vi "Cache Message.vi"(10 "Message":T1={"Source"="", "Destination"="", "Time Stamp"=timestamp(0 s since 1904-01-01), "Command"="", "Data"=variant(string "")}, 11 "Message History In":string[][](array[string])) -> (3 "Message History Out":string[][](array[string]))   [LabVIEW 2020, in "RxnRover.lvlib"]
uses:
  RxnRover.lvlib
  <userlib>/RxnRover/DynamicReentrant/src/Type Defs/Message.ctl
  <userlib>/RxnRover/DynamicReentrant/Dynamic Reentrant.lvlib
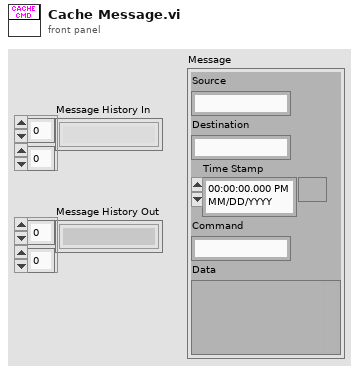
[diagram p1: front panel]
types:
  T1 = typedef "Dynamic Reentrant.lvlib/Message.ctl" = cluster{"Source":string, "Destination":string, "Time Stamp":timestamp, "Command":string, "Data":variant}
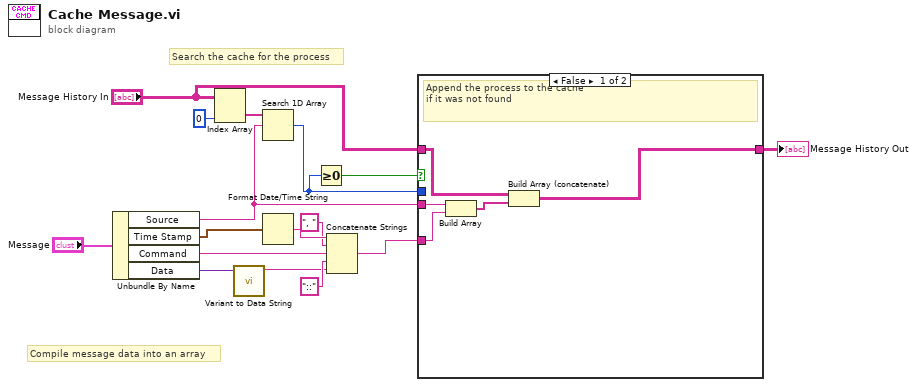
[diagram p0: block diagram]
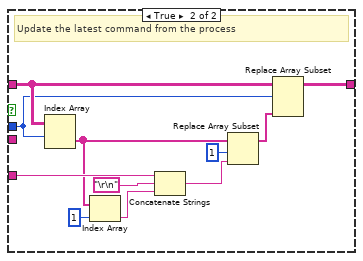
[diagram p2: hidden frame]
diagram:
  # "Search the cache for the process"
  # "Compile message data into an array"
  n1 = Unbundle By Name("Message") -> ("Source"=w3:string, "Time Stamp"=w9:timestamp, "Command"=w8:string, "Data"=w1:variant)
  n2 = Index Array(array="Message History In", index (col)=0 ("disabled index (col)")) -> (element=w16:string[])  [unwired: 1 in]
  n3 = call "Variant to Data String.vi"("Data"=w1) -> ("string"=w2:string)  [unwired: 9 in, 1 out]
  n4 = Search 1D Array(1D array=w16, element=w3) -> (index of element=w10:i32)  [unwired: 1 in]
  n5 = Format Date/Time String(seconds (now)=w9) -> (date/time string=w7:string)  [unwired: 2 in]
  n6 = Greater Or Equal To 0?(x=w10) -> (x >= 0?=w14:bool)
  n7 = Concatenate Strings(w7, ", " ("string"), w8, "::" ("string"), w2) -> (w4:string)
  n8 = case shown="False" w14 {
    tunnel: w10 -> [_ w27]
    tunnel: [w20 w26] -> w12
    tunnel: "Message History In" -> [w21 w28]
    tunnel: w4 -> [w18 w30]
    tunnel: w3 -> [w19 _]
    frame False {
      # "Append the process to the cache\nif it was not found"
      n9 = Build Array(w19, w18) -> (w17:string[])
      n10 = Build Array (concatenate)(w21, w17) -> (w20:string[][])
    }
    frame True {
      # "Update the latest command from the process"
      n11 = Index Array(array=w28, index (row)=w27) -> (element=w25:string[])  [unwired: 1 in]
      n12 = Index Array(array=w25, index=1) -> (element=w31:string)
      n13 = Concatenate Strings(w30, "\r\n", w31) -> (w23:string)
      n14 = Replace Array Subset(array=w25, new element=w23, index=1) -> (w22:string[])
      n15 = Replace Array Subset(array=w28, new element=w22, index (row)=w27) -> (w26:string[][])  [unwired: 1 in]
    }
  }
  "Message History Out" <- w12
